vi "add_CameraOpen.vi"(4 "Camera Settings":T1={"Camera Name"="1", "FPS"=20.0, "Camera Controls"=[], "Resolution"=enum."(1280, 800)"}, 5 "msg in":string) -> (2 "msg out":string)   [LabVIEW 2015]
uses:
  std_msgs/subs/stringScalar.vi
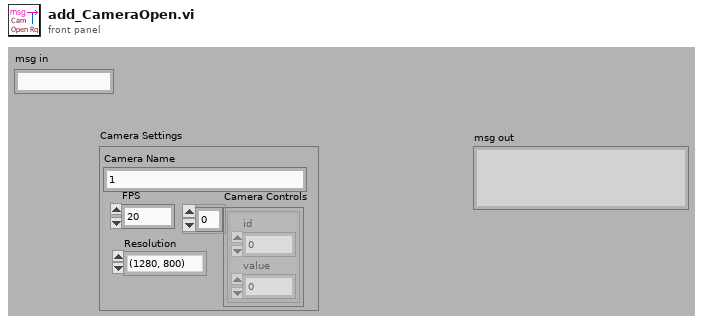
[diagram p1: front panel]
types:
  T1 = cluster{"Camera Name":string, "FPS":sgl, "Camera Controls":cluster{"id":i32, "value":i32}[], "Resolution":enum16{"(1280, 800)", "(960, 600)", "(640, 400)", "(480, 300)", "(384, 240)", "(320, 200)"}}
  T2 = cluster{"FPS":sgl, "Camera Controls":cluster{"id":i32, "value":i32}[], "Width":i32, "Height":i32}
  T3 = enum16{"(1280, 800)", "(960, 600)", "(640, 400)", "(480, 300)", "(384, 240)", "(320, 200)"}
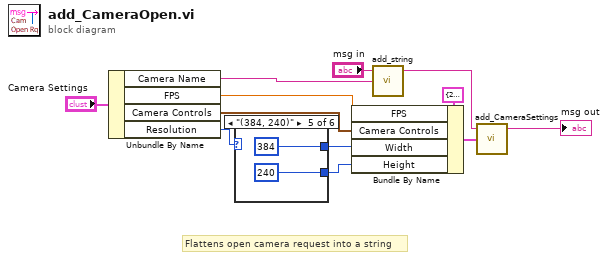
[diagram p0: block diagram]
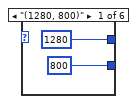
[diagram p2: hidden frame]
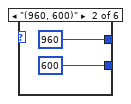
[diagram p3: hidden frame]
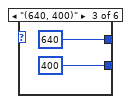
[diagram p4: hidden frame]
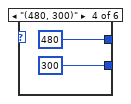
[diagram p5: hidden frame]
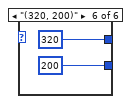
[diagram p6: hidden frame]
diagram:
  # "Flattens open camera request into a string"
  n1 = Unbundle By Name("Camera Settings") -> ("Camera Name"=w11:string, "FPS"=w8:sgl, "Camera Controls"=w7:cluster{"id":i32, "value":i32}[], "Resolution"=w10:T3)
  n2 = case shown="\"(384, 240)\"" w10 {
    tunnel: [1280 960 640 480 384 320] -> w6
    tunnel: [800 600 400 300 240 200] -> w5
    frame "(1280, 800)" {
    }
    frame "(960, 600)" {
    }
    frame "(640, 400)" {
    }
    frame "(480, 300)" {
    }
    frame "(384, 240)" {
    }
    frame "(320, 200)" {
    }
  }
  n3 = Bundle By Name(cluster=T2 {"FPS"=20.0, "Camera Controls"=[], "Width"=0, "Height"=0} ("Camera Settings"), "FPS"=w8, "Camera Controls"=w7, "Width"=w6, "Height"=w5) -> (w4:T2)
  n4 = call-poly "add_string.vi"("String"=w11, "msg in"="msg in") -> ("msg out"=w3:string)  [unwired: 3 in]
  n5 = call "add_CameraSettings.vi"("Camera Settings"=w4, "msg in"=w3) -> ("msg out"=→"msg out":string)  [unwired: 3 in]
